vi "Read State_.vi"(11 "Model in":refnum<class "Model.lvclass">) -> (2 "state:":T1=enum."EndingCycleState", 3 "Model out":refnum<class "Model.lvclass">)   [LabVIEW 2013, in "Model.lvclass"]
uses:
  Model.lvclass
  Typedefs/StateSelector.ctl
  Model.lvclass/Model.ctl
  Typedefs/AITDTTypedefs.lvlib
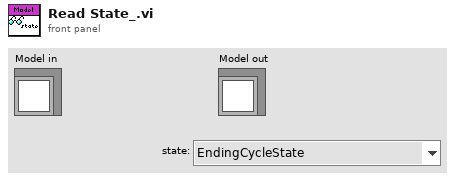
[diagram p1: front panel]
types:
  T1 = typedef "AITDTTypedefs.lvlib/StateSelector.ctl" = enum16{"AwaitingSetpointAcknowledgmentState", "EndingCycleState", "FaultState", "OffState", "PausingState", "RequestingNewSetpointState", "SamplingState", "SettlingState", "SoakingState", "StabilizingState", "StandbyState", "StoppedState", "TransitioningTemperatureState"}
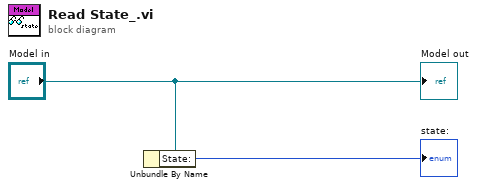
[diagram p0: block diagram]
diagram:
  n1 = Unbundle By Name("Model in") -> ("State:"=→"state:":T1)
  "Model out" <- "Model in"
